vi "Data e ora.vi"() -> (0 "Data_ora_txt":string, 1 "date_ora":string)   [LabVIEW 2012]
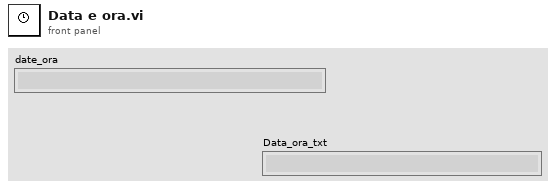
[diagram p1: front panel]
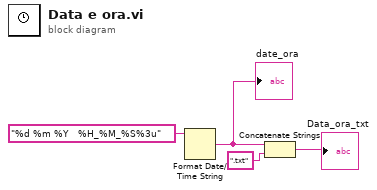
[diagram p0: block diagram]
diagram:
  n1 = Format Date/Time String(time format string (%c)="%d %m %Y   %H_%M_%S%3u") -> (date/time string=w1:string)  [unwired: 2 in]
  "date_ora" <- w1
  n2 = Concatenate Strings(w1, ".txt" ("string")) -> (→"Data_ora_txt":string)
